vi "VCS Analog Output Configuration.vi"(0 "axis in":cluster{"keyHandle":u32, "nodeId":u16}={"keyHandle"=0, "nodeId"=1}, 7 "configuration":T1={"analogOutuptNumber"=1, "configuration"=0} {"configuration" items=["general purpose A", "general purpose B"]}, 11 "error in (no error)":errorcluster) -> (4 "axis out":cluster{"keyHandle":u32, "nodeId":u16}={"keyHandle"=0, "nodeId"=1}, 15 "error out":errorcluster)   [LabVIEW 2017, in "maxonEPOS.lvlib"]
doc: "<B>VCS_AnalogInputConfiguration</B> sets parameter for one analog input."
uses:
  Examples/maxonEPOS.lvlib
  SSI_Tool/InstrumentsInterfaces/Motordriver/maxon EPOS/Resources/EposCmd64.dll
  Resources/EposCmd.dll
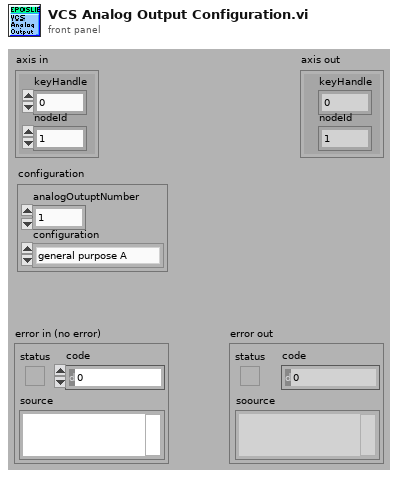
[diagram p1: front panel]
types:
  T1 = cluster{"analogOutuptNumber":u16, "configuration":u16}
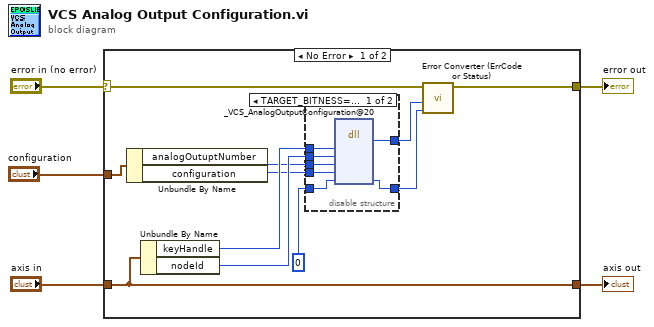
[diagram p0: block diagram]
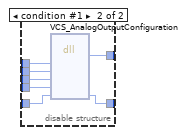
[diagram p2: hidden frame]
diagram:
  n1 = case shown="No Error" "error in (no error)" {
    selector: "error in (no error)" -> [w14 w31]
    tunnel: "axis in" -> [w16 w32]
    tunnel: [w16 w32] -> w4
    tunnel: [w15 w31] -> w3
    tunnel: "configuration" -> [w8 _]
    frame No Error {
      n2 = Unbundle By Name(w8) -> ("analogOutuptNumber"=w7:u16, "configuration"=w6:u16)
      n3 = Unbundle By Name(w16) -> ("keyHandle"=w11:u32, "nodeId"=w12:u16)
      n4 = disable-structure shown="TARGET_BITNESS==32, Standard" {
        disable-tunnel: u32 0 ("pErrorCode") -> [w23 w30]
        disable-tunnel: w12 -> [w22 w29]
        disable-tunnel: w11 -> [w21 w28]
        disable-tunnel: [w20 w27] -> w10
        disable-tunnel: [w19 w26] -> w9
        disable-tunnel: w7 -> [w18 w25]
        disable-tunnel: w6 -> [w17 w24]
        frame condition #0 (active) {
          n5 = dll-call lib="C:/workspace/project/scancon/sw/SSI_Tool/InstrumentsInterfaces/Motordriver/maxon EPOS/Resources/EposCmd.*" fn="_VCS_AnalogOutputConfiguration@20" ("EposCmd.dll:_VCS_AnalogInputConfiguration@24")("KeyHandle"=w21, "NodeId"=w22, "AnlogOutputNb"=w18, "Configuration"=w17, "pErrorCode"=w23) -> ("Rückgabetyp"=w20:i32, "pErrorCode"=w19:u32)  [unwired: 7 in, 2 out]
        }
        frame condition #1 {
          n6 = dll-call lib="C:/Sources/LabView/maxon EPOS/Resources/EposCmd64.*" fn="VCS_AnalogOutputConfiguration" ("EposCmd.dll:_VCS_AnalogInputConfiguration@24")("KeyHandle"=w28, "NodeId"=w29, "AnlogOutputNb"=w25, "Configuration"=w24, "pErrorCode"=w30) -> ("Rückgabetyp"=w27:i32, "pErrorCode"=w26:u32)  [unwired: 7 in, 2 out]
        }
      }
      n7 = call "Error Converter (ErrCode or Status).vi"("error code"=w9, "return type"=w10, "error in (no error)"=w14) -> ("error out"=w15:errorcluster)  [unwired: 7 in]
    }
    frame Error {
    }
  }
  "error out" <- w3
  "axis out" <- w4
